vi "ExSetTemperature.vi"(1 "error in (no error)":errorcluster) -> (0 "error out":errorcluster)   [LabVIEW 2010]
uses:
  Open-Close Hardware/CamHandle.vi
panel:
  in  "Temperature":dbl=-10.0 format="%.2f"
  # "ExSetTemperature.vi : set the desired temperature then run VI"
  # "Note : Most cameras have an optimized \ndefault temperature. By changing the \ntemperature from the default the camera\nmay not perform to it's best. Please \ncontact camera manufacurer if you \nthink the default should not be used."
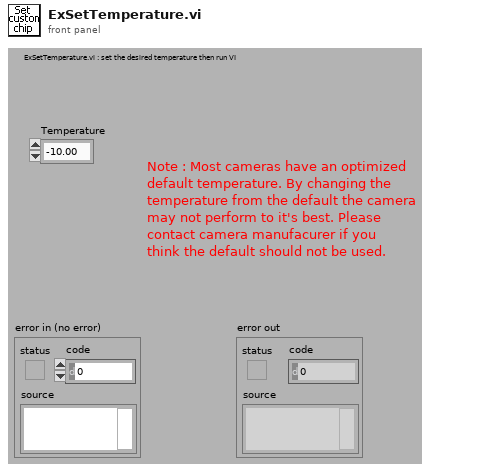
[diagram p1: front panel]
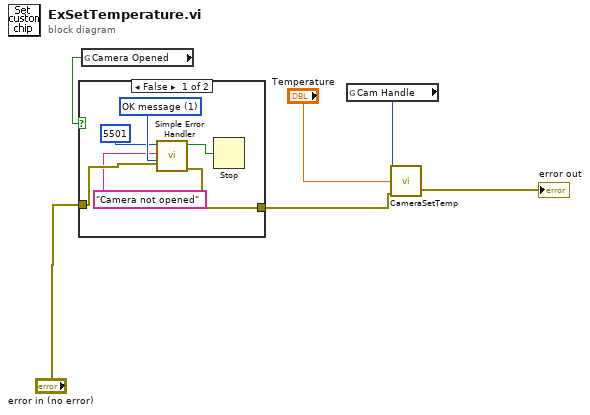
[diagram p0: block diagram]
diagram:
  n1 = global read "CamHandle.vi" "Camera Opened"() -> (w6:bool)
  n2 = case shown="False" w6 {
    tunnel: "error in (no error)" -> [w11 w13]
    tunnel: [w10 w13] -> w4
    frame False {
      w12 = u16 1 items=["no dialog", "OK message", "continue or stop message"] ("type of dialog (OK msg:1)")
      n3 = call <vilib>:"Simple Error Handler.vi"("error code (no error:0)"=5501, "error source (\" \")"="Camera not opened", "type of dialog (OK msg:1)"=w12, "error in (no error)"=w11) -> ("error?"=w8:bool, "error out"=w10:errorcluster)  [unwired: 1 in, 3 out]
      n4 = Stop(stop? (T)=w8) -> ()
    }
    frame True {
    }
  }
  n5 = global read "CamHandle.vi" "Cam Handle"() -> (w1:u32)
  n6 = call <userlib>:"CameraSetTemp.vi"("error in (no error)"=w4, "Temperature"="Temperature", "Camera Handle"=w1) -> ("error out"=→"error out":errorcluster)  [unwired: 1 out]
